vi "Aplicatie proiect.vi"() -> ()   [LabVIEW 2022 SP3]
uses:
  <vilib>/MakerHub/LINX/Public/Peripherals/PWM/PWM Set Duty Cycle 1 Chan.vi
  <vilib>/MakerHub/LINX/Public/Utilities/Open Serial.vi
  <vilib>/MakerHub/LINX/Public/Peripherals/PWM/PWM Set Duty Cycle N Chans.vi
  <vilib>/MakerHub/LINX/LMH-LINX.lvlib
panel:
  in  "Digital Output Channel":u8=13
  in  "Serial Port":refnum<visa-resource-name>
  in  "Stop Button":bool
  in  "Temperatura dorita":dbl
  out "Tensiune electrica necesara":dbl
  out "Factor de umplere optim":dbl
  # "Tabele de cautare"
  # "[grade C]"
  # "[V]"
  # "[%]"
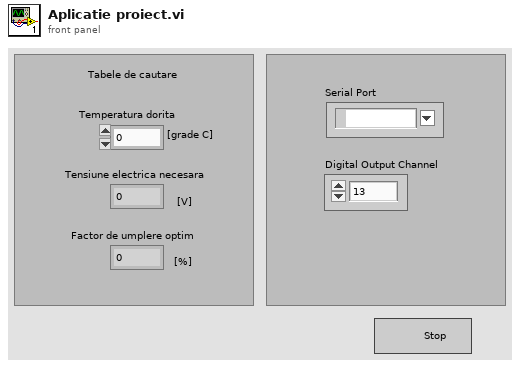
[diagram p1: front panel]
types:
  T1 = typedef "LMH-LINX.lvlib/LINX Ref.ctl" = cluster{"IO":T2, "Interface":T3, "LINX Device Config":T4}
  T2 = typedef "LMH-LINX.lvlib/Platform.ctl" = enum16{"Remote", "Local"}
  T3 = typedef "LMH-LINX.lvlib/Interface.ctl" = enum16{"Serial", "TCP"}
  T4 = typedef "LMH-LINX.lvlib/Device.lvlib/LINX Device Config.ctl" = cluster{"Interface":T3, "COM Port":refnum<visa-resource-name>, "TCP Configuration":T5, "Device Family":u8, "Device ID":u8, "Device Name":string, "TCP Ref":refnum<k5>, "Channels":T6}
  T5 = typedef "LMH-LINX.lvlib/Device.lvlib/TCP Config.ctl" = cluster{"IP Address":string, "Port":u16}
  T6 = typedef "LMH-LINX.lvlib/Channels.ctl" = cluster{"DI":u8[], "DO":u8[], "AI":u8[], "AO":u8[], "PWM":u8[], "QE":u8[], "UART":u8[], "I2C 2":u8[], "SPI":u8[], "CAN":u8[], "Servo":u8[], "AI Ref (V)":dbl, "AI Resolution (Bits)":u8, "AO Ref (V)":dbl, "AO Resolution (Bits)":u8}
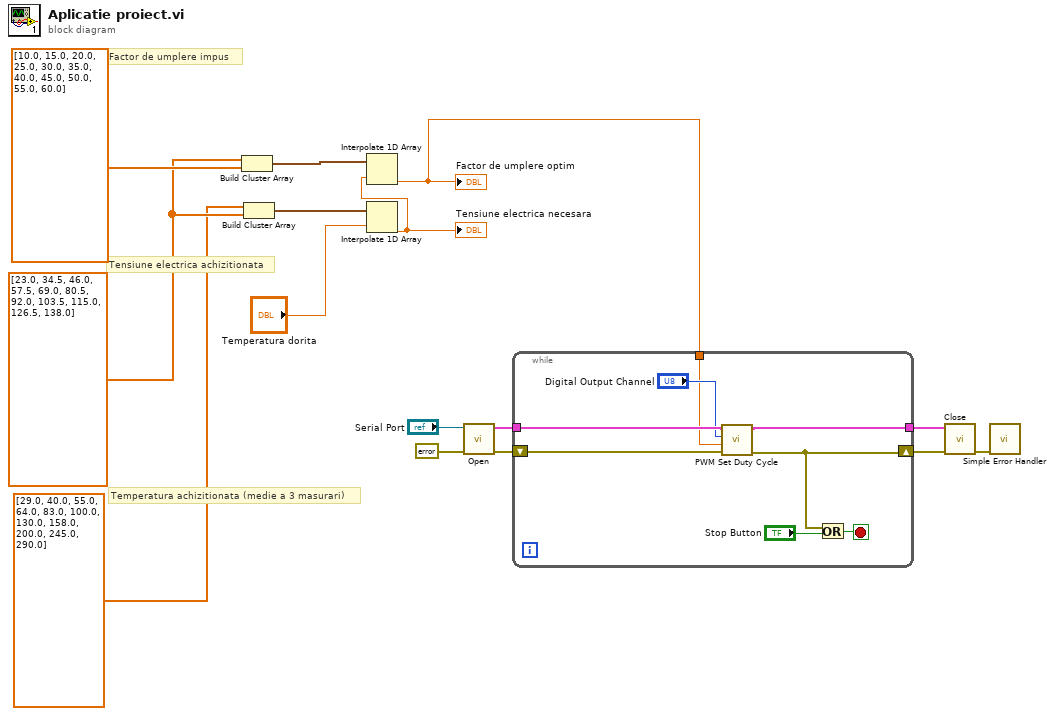
[diagram p0: block diagram]
diagram:
  w11 = dbl[] [23.0, 34.5, 46.0, 57.5, 69.0, 80.5, 92.0, 103.5, 115.0, 126.5, 138.0] ("array of numbers or points")
  # "Temperatura achizitionata (medie a 3 masurari)"
  # "Tensiune electrica achizitionata"
  # "Factor de umplere impus"
  n1 = Build Cluster Array(w11, dbl[] [10.0, 15.0, 20.0, 25.0, 30.0, 35.0, 40.0, 45.0, 50.0, 55.0, 60.0] ("array of numbers or points")) -> (w14:cluster{dbl, dbl}[])
  n2 = Build Cluster Array(dbl[] [29.0, 40.0, 55.0, 64.0, 83.0, 100.0, 130.0, 158.0, 200.0, 245.0, 290.0] ("array of numbers or points"), w11) -> (w15:cluster{dbl, dbl}[])
  n3 = Interpolate 1D Array(1:"Temperatura dorita", 2:w15) -> (0:w13:dbl)
  "Tensiune electrica necesara" <- w13
  n4 = Interpolate 1D Array(1:w13, 2:w14) -> (0:w1:dbl)
  "Factor de umplere optim" <- w1
  n5 = call-poly <vilib>:"Open.vi"("Error In"=errorcluster {"status"=FALSE, "code"=0, "source"=""}, "Serial Port"="Serial Port") -> ("Error Out"=w7:errorcluster, "LINX Resource"=w8:T1)  [unwired: 7 in, 1 out]
  n6 = while {
    tunnel: w8 -> [w21]
    tunnel: [w20] -> w6
    shift-right: [w18] -> w5
    shift-left: w7 -> [w19]
    tunnel: w1 -> [w16]
    stop <- w23 stop-if-true
    n7 = call-poly <vilib>:"PWM Set Duty Cycle.vi"("Error In"=w19, "Duty Cycle (0-1)"=w16, "PWM Channel"="Digital Output Channel", "LINX Resource"=w21) -> ("Error Out"=w18:errorcluster, "LINX Resource"=w20:T1)  [unwired: 6 in]
    n8 = Or(x=w18, y="Stop Button") -> (x .or. y?=w23:bool)
  }
  n9 = call <vilib>:"Close.vi"("Error In"=w5, "LINX Resource"=w6) -> ("Error Out"=w3:errorcluster)  [unwired: 9 in]
  n10 = call <vilib>:"Simple Error Handler.vi"("error in (no error)"=w3) -> ()  [unwired: 4 in, 5 out]
